vi "Select.vi"(6 "Table Name":string, 7 "condition":string, 8 "error in (no error)":errorcluster, 10 "Selected ColumnName List":variant, 11 "DataBase_SQL in":refnum<class "DataBase_SQL.lvclass">) -> (0 "error out":errorcluster, 1 "FirstRow":string[](array[string]), 2 "Datas":string[][](table), 3 "DataBase_SQL out":refnum<class "DataBase_SQL.lvclass">, 4 "SQL Query":string)   [LabVIEW 2021, in "DataBase_SQL.lvclass"]
uses:
  <userlib>/John_Lib/DataBase/DataBase_SQL/DataBase_SQL.lvclass
  eba593ed-bd29-4c09-bdf8-b691de92e928.vi
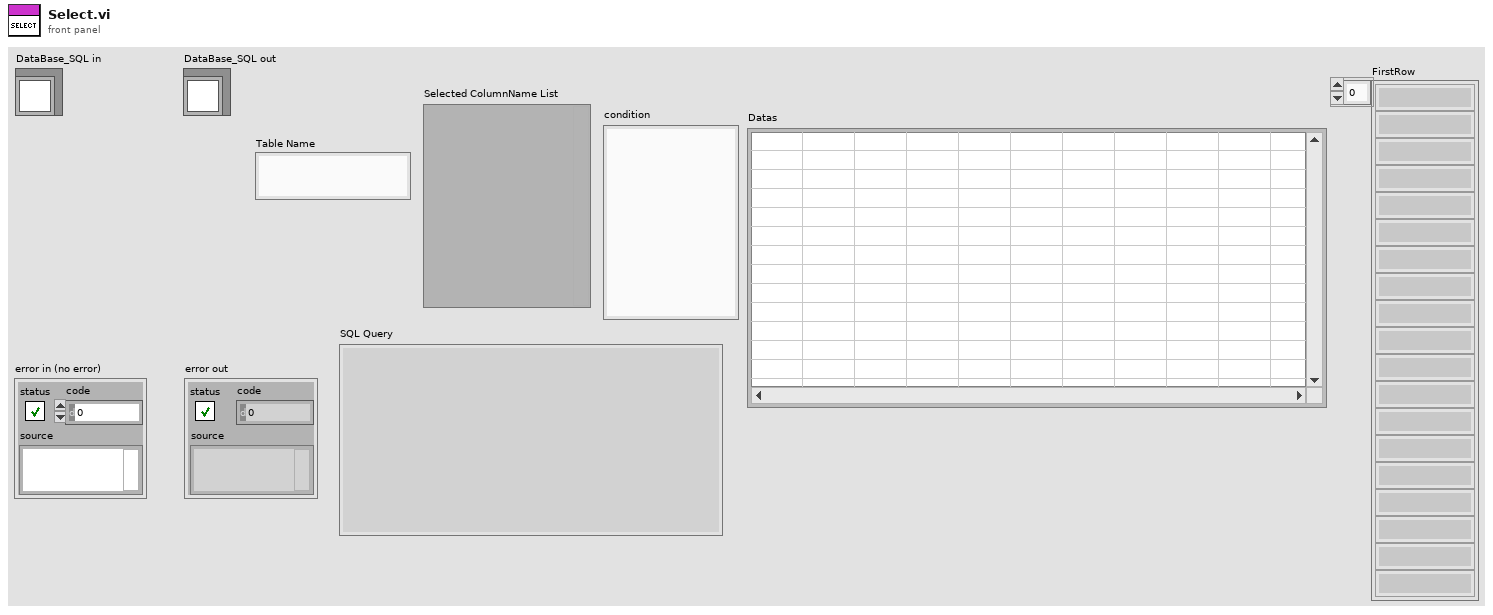
[diagram p1: front panel]
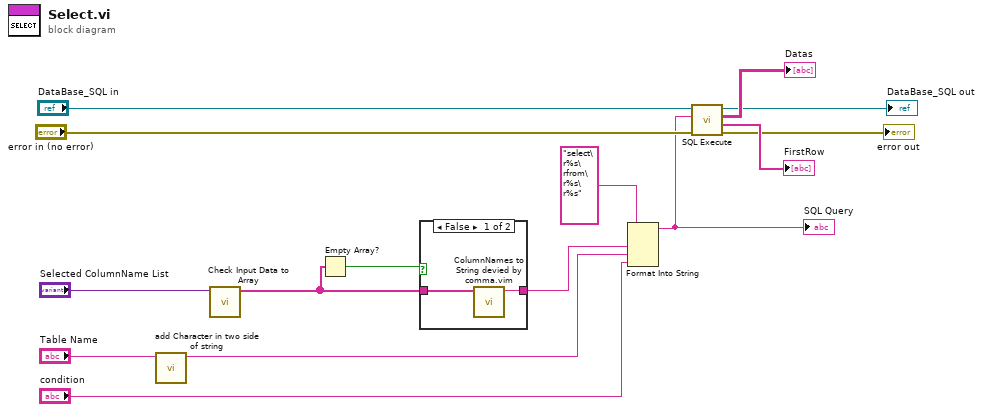
[diagram p0: block diagram]
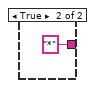
[diagram p2: hidden frame]
diagram:
  n1 = call <userlib>:"add Character in two side of string.vi"("Sting In"="Table Name") -> ("String Out"=w1:string)  [unwired: 10 in]
  n2 = call <userlib>:"Check Input Data to Array.vi"("String Array/ String"="Selected ColumnName List") -> ("ColumnsNameList"=w3:string[])  [unwired: 9 in, 1 out]
  n3 = Empty Array?(array=w3) -> (empty?=w2:bool)
  n4 = case shown="False" w2 {
    tunnel: [w17 "*" ("Columns,String")] -> w13
    tunnel: w3 -> [w16 _]
    frame False {
      n5 = call "ColumnNames to String devied by comma.vim"("ColumnNames"=w16) -> ("Columns,String"=w17:string)  [unwired: 10 in]
    }
    frame True {
    }
  }
  n6 = Format Into String(format string="select\r%s\rfrom\r%s\r%s", w13, w1, "condition") -> (resulting string=w5:string)  [unwired: 2 in, 1 out]
  "SQL Query" <- w5
  n7 = call-dynamic "SQL Execute.vi"("error in (no error)"="error in (no error)", "Command Text"=w5, "DataBase_SQL in"="DataBase_SQL in") -> ("error out"=→"error out":errorcluster, "FirstRow"=→"FirstRow":string[], "Datas"=→"Datas":string[][], "DataBase_SQL out"=→"DataBase_SQL out":refnum<class "DataBase_SQL.lvclass">)  [unwired: 4 in, 1 out]
